vi "Generate Comments.vi"(7 "error in (no error)":errorcluster, 9 "cluster":T1) -> (0 "error out":errorcluster, 3 "Comments":string)   [LabVIEW 2016, in "Control Experiment.lvclass"]
uses:
  Control Experiment.lvclass
  Typedefs/Comments-cluster.ctl
  <userlib>/LevyLab/Krohn Hite 7008/typedefs/Gain-Enum.ctl
  <userlib>/LevyLab/Krohn Hite 7008/typedefs/Shunt-Enum.ctl
  <userlib>/LevyLab/Krohn Hite 7008/KH7008.lvclass
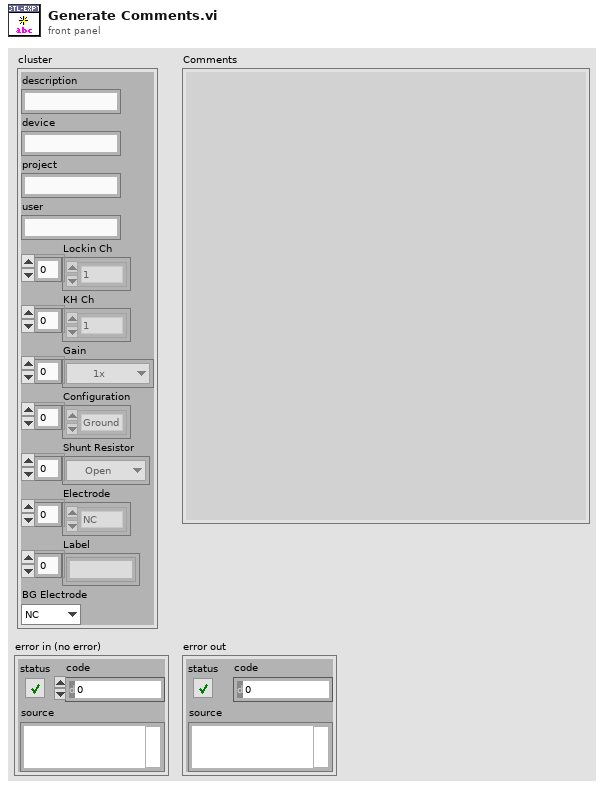
[diagram p1: front panel]
types:
  T1 = typedef "Control Experiment.lvclass/Comments-cluster.ctl" = cluster{"description":string, "device":string, "project":string, "user":string, "Lockin Ch":enum16{"1", "2", "3", "4", "5", "6", "7", "8"}[], "KH Ch":enum16{"1", "2", "3", "4", "5", "6", "7", "8"}[], "Gain":T2[], "Configuration":enum16{"Ground", "Current", "Voltage", "Gate"}[], "Shunt Resistor":T3[], "Electrode":enum16{"NC", "26", "27", "28", "1", "2", "3", "4", "5", "6", "7", "8", "9", "10", "11", "12", "13", "14", "15", "16", "17", "18", "19", "20", "21", "22", "23", "24", "25"}[], "Label":string[], "BG Electrode":enum16{"NC", "26", "27", "28", "1", "2", "3", "4", "5", "6", "7", "8", "9", "10", "11", "12", "13", "14", "15", "16", "17", "18", "19", "20", "21", "22", "23", "24", "25"}}
  T2 = typedef "KH7008.lvclass/Gain-Enum.ctl" = enum16{"1x", "10x", "100x", "1000x"}
  T3 = typedef "KH7008.lvclass/Shunt-Enum.ctl" = enum16{"Open", "50 Ohms", "500 Ohms", "5k Ohms", "50k Ohms"}
  T4 = enum16{"NC", "26", "27", "28", "1", "2", "3", "4", "5", "6", "7", "8", "9", "10", "11", "12", "13", "14", "15", "16", "17", "18", "19", "20", "21", "22", "23", "24", "25"}[]
  T5 = enum16{"NC", "26", "27", "28", "1", "2", "3", "4", "5", "6", "7", "8", "9", "10", "11", "12", "13", "14", "15", "16", "17", "18", "19", "20", "21", "22", "23", "24", "25"}
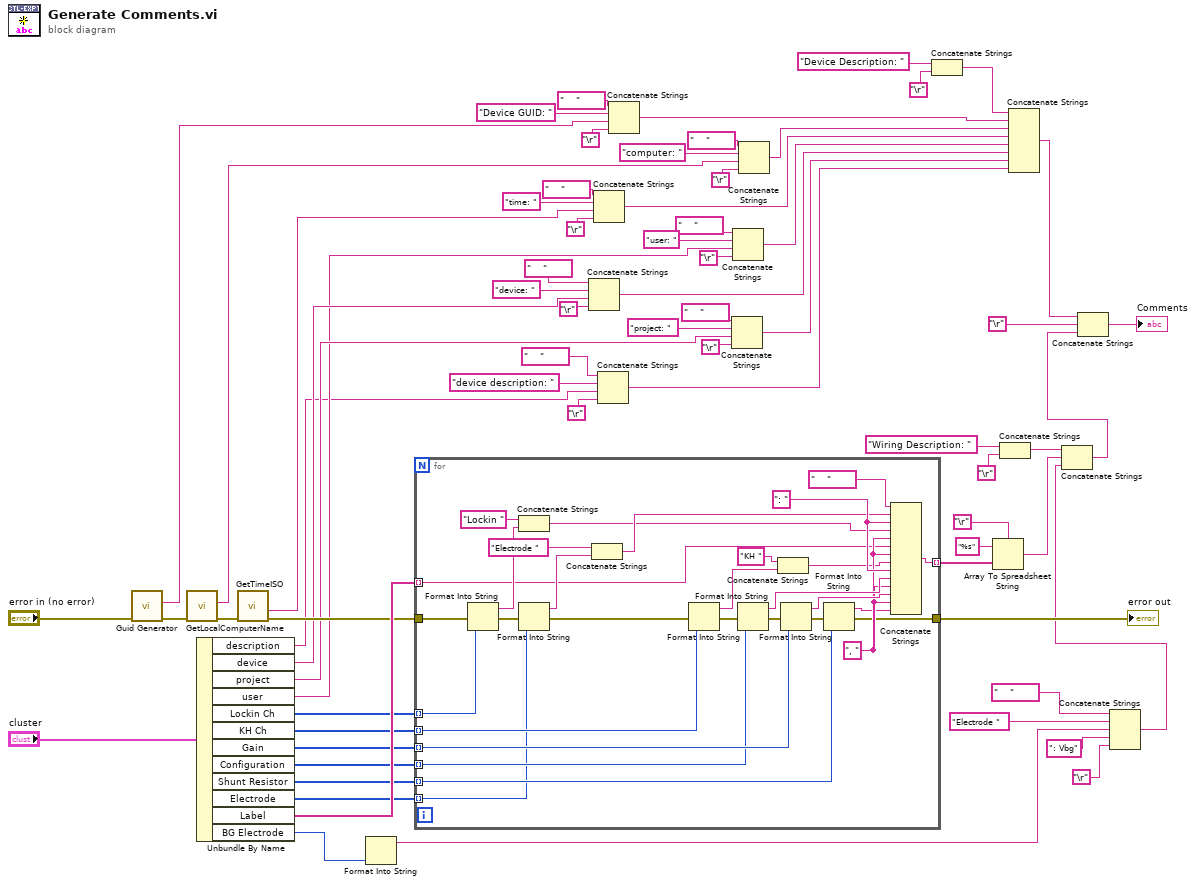
[diagram p0: block diagram]
diagram:
  n1 = call <vilib>:"Guid Generator.vi"("error in (no error)"="error in (no error)") -> ("error out"=w42:errorcluster, "GUID"=w26:string)  [unwired: 9 in]
  n2 = call <userlib>:"GetLocalComputerName.vi"("error in (no error)"=w42) -> ("error out"=w38:errorcluster, "Name"=w22:string)  [unwired: 9 in]
  n3 = Unbundle By Name("cluster") -> ("description"=w40:string, "device"=w49:string, "project"=w48:string, "user"=w47:string, "Lockin Ch"=w63:enum16{"1", "2", "3", "4", "5", "6", "7", "8"}[], "KH Ch"=w64:enum16{"1", "2", "3", "4", "5", "6", "7", "8"}[], "Gain"=w65:T2[], "Configuration"=w66:enum16{"Ground", "Current", "Voltage", "Gate"}[], "Shunt Resistor"=w67:T3[], "Electrode"=w68:T4, "Label"=w69:string[], "BG Electrode"=w8:T5)
  n4 = call "GetTimeISO.vi"("error in (no error)"=w38) -> ("error out"=w57:errorcluster, "ISO 8601 date-time string"=w41:string)  [unwired: 8 in, 1 out]
  n5 = Format Into String(w8) -> (resulting string=w6:string)  [unwired: 3 in, 1 out]
  n6 = for {
    tunnel: w63 -> [w71] mode=indexing
    tunnel: w64 -> [w73] mode=indexing
    tunnel: w65 -> [w75] mode=indexing
    tunnel: w66 -> [w74] mode=indexing
    tunnel: w67 -> [w76] mode=indexing
    tunnel: w68 -> [w72] mode=indexing
    tunnel: w69 -> [w78] mode=indexing
    tunnel: [w96] -> w58 mode=indexing
    tunnel: w57 -> [w86]
    tunnel: [w81] -> w56
    w91 = ", "
    w94 = ": "
    n7 = Format Into String(error in=w86, w71) -> (resulting string=w98:string, error out=w85:errorcluster)  [unwired: 2 in]
    n8 = Concatenate Strings("Lockin ", w98) -> (w79:string)
    n9 = Format Into String(error in=w85, w72) -> (resulting string=w95:string, error out=w77:errorcluster)  [unwired: 2 in]
    n10 = Concatenate Strings("Electrode ", w95) -> (w80:string)
    n11 = Format Into String(error in=w77, w73) -> (resulting string=w87:string, error out=w84:errorcluster)  [unwired: 2 in]
    n12 = Format Into String(error in=w84, w74) -> (resulting string=w93:string, error out=w83:errorcluster)  [unwired: 2 in]
    n13 = Concatenate Strings("KH ", w87) -> (w88:string)
    n14 = Format Into String(error in=w83, w75) -> (resulting string=w92:string, error out=w82:errorcluster)  [unwired: 2 in]
    n15 = Format Into String(error in=w82, w76) -> (resulting string=w90:string, error out=w81:errorcluster)  [unwired: 2 in]
    n16 = Concatenate Strings("    " ("string"), w80, w94, w79, w91, w78, w91, w88, w94, w93, w91, w92, w91, w90) -> (w96:string)
  }
  "error out" <- w56
  n17 = Concatenate Strings("    " ("string"), "device: " ("string"), w49, "\r") -> (w17:string)
  n18 = Concatenate Strings("    " ("string"), "time: " ("string"), w41, "\r") -> (w19:string)
  n19 = Concatenate Strings("    " ("string"), "device description: " ("string"), w40, "\r") -> (w15:string)
  n20 = Concatenate Strings("    " ("string"), "Device GUID: " ("string"), w26, "\r") -> (w21:string)
  n21 = Concatenate Strings("    " ("string"), "project: " ("string"), w48, "\r") -> (w16:string)
  n22 = Concatenate Strings("    " ("string"), "user: " ("string"), w47, "\r") -> (w18:string)
  n23 = Concatenate Strings("    " ("string"), "computer: " ("string"), w22, "\r") -> (w20:string)
  n24 = Concatenate Strings("Device Description: " ("string"), "\r") -> (w30:string)
  n25 = Array To Spreadsheet String(delimiter (Tab)="\r", array=w58, 3:"%s" ("format string")) -> (spreadsheet string=w10:string)
  n26 = Concatenate Strings("Wiring Description: " ("string"), "\r") -> (w11:string)
  n27 = Concatenate Strings(w30, w21, w20, w19, w18, w17, w16, w15) -> (w14:string)
  n28 = Concatenate Strings("    " ("string"), "Electrode ", w6, ": Vbg", "\r") -> (w3:string)
  n29 = Concatenate Strings(w11, w10, w3) -> (w9:string)
  n30 = Concatenate Strings(w14, "\r", w9) -> (→"Comments":string)
